vi "Add Tag.vi"(8 "error in":errorcluster, 11 "references":T1) -> (0 "error out":errorcluster, 2 "newtag?":bool)   [LabVIEW 2013, in "Shared Memory Editor Node.lvclass"]
doc: "Copyright 2016 National Instruments Corporation\n\nLicensed under the Apache License, Version 2.0 (the \"License\"); you may not use this file except in compliance with the License. You may obtain a copy of the License at http://www.apache.org/licenses/LICENSE-2.0\nUnless required by applicable law or agreed to in writing, software distributed under the License is distributed on an \"AS IS\" BASIS, WITHOUT WARRANTIES OR CONDITIONS OF ANY KIND, either express or implied. See the License for the specific language governing permissions and limitations under the License."
uses:
  Shared Memory Editor Node.lvclass
  <vilib>/NI/DCAF Table API/Table Manager/object ref.ctl
  <vilib>/NI/DCAF/Tag Editor Core/Configuration Editor/Classes/Engine Parent/Engine Parent Editor Node.lvclass
  <vilib>/NI/DCAF/Tag Editor Core/Configuration Editor/Classes/Module editor node/module editor node.lvclass
  module/configuration/Shared Memory Configuration.lvclass
  <vilib>/NI/DCAF Table API/Table Manager/Table Manager.lvclass
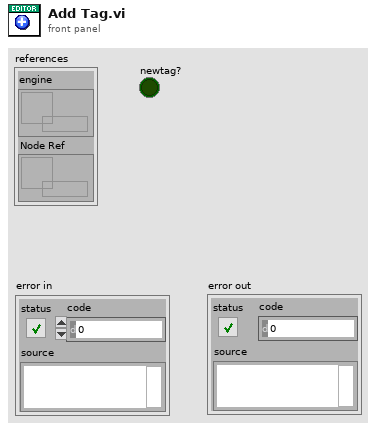
[diagram p1: front panel]
types:
  T1 = typedef "Table Manager.lvlib/Table Manager.lvclass/object ref.ctl" = cluster{"engine":refnum<data-value>, "Node Ref":refnum<data-value>}
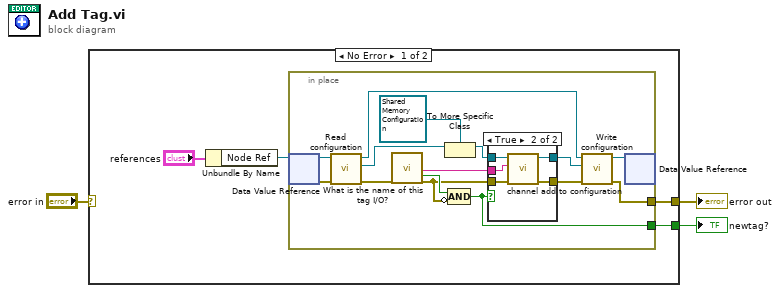
[diagram p0: block diagram]
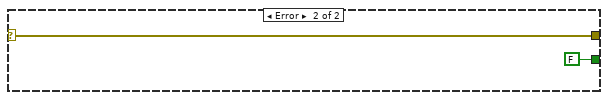
[diagram p3: hidden frame]
diagram:
  n1 = case shown="No Error" "error in" {
    selector: "error in" -> [_ w31]
    tunnel: [w7 w31] -> w3
    tunnel: [w4 FALSE] -> w1
    frame No Error {
      n2 = Unbundle By Name("references") -> ("Node Ref"=w5:refnum<data-value>)
      n3 = in-place {
        in-place-border: [w10] -> w7
        in-place-border: [w22] -> w4
        n4 = in-place-dvr #1(w5) -> (w15:refnum<class "module editor node.lvclass">, w9:errorcluster)
        n5 = call-dynamic "Read configuration.vi"("error in"=w9, "NISE_CEF_serializable node in"=w15) -> ("error out"=w8:errorcluster, "configuration"=w14:refnum<class "NISE_CEF_serializable configuration.lvclass">, "NISE_CEF_serializable node out"=w16:refnum<class "module editor node.lvclass">)  [unwired: 7 in]
        n6 = call "What is the name of this tag I/O?"("error in (no error)"=w8) -> ("Tag Name"=w19:string, "OK"=w21:bool, "error out"=w20:errorcluster)  [unwired: 16 in]
        n7 = To More Specific Class(target class=refnum<class "Shared Memory Configuration.lvclass"> refnum ("tag select module configuration in"), reference=w14) -> (specific class reference=w18:refnum<class "Shared Memory Configuration.lvclass">)  [unwired: 1 in, 1 out]
        n8 = Compound Arithmetic op=AND(w21, invert w20) -> (w22:bool)
        n9 = case shown="True" w22 {
          tunnel: w20 -> [w23 w28]
          tunnel: [w24 w27] -> w13
          tunnel: w18 -> [w24 w29]
          tunnel: [w23 w25] -> w11
          tunnel: w19 -> [_ w26]
          frame False {
          }
          frame True {
            n10 = call "channel add to configuration.vi"("error in"=w28, "channel name"=w26, "shared memory module configuration in"=w29) -> ("error out"=w25:errorcluster, "shared memory module configuration out"=w27:refnum<class "Shared Memory Configuration.lvclass">)  [unwired: 6 in, 1 out]
          }
        }
        n11 = call-dynamic "Write configuration.vi"("error in"=w11, "configuration"=w13, "NISE_CEF_serializable node in"=w16) -> ("error out"=w10:errorcluster, "NISE_CEF_serializable node out"=w12:refnum<class "module editor node.lvclass">)  [unwired: 7 in]
        n12 = in-place-dvr #1(w12) -> ()  [unwired: 2 out]
      }
    }
    frame Error {
    }
  }
  "error out" <- w3
  "newtag?" <- w1
